vi "Results.vi"(0 "Code":dbl format="%#_12g", 5 "Voltage":dbl format="%#_12g", 11 "Error In":errorcluster, 12 "Slope":dbl format="%#_12g", 13 "Offset_Error":dbl format="%#_12g", 14 "Gain_error":dbl format="%#_12g") -> (15 "error out":errorcluster)   [LabVIEW 2019]
uses:
  common/Comman_nilesh/File_Write/Data_Logging.lvclass
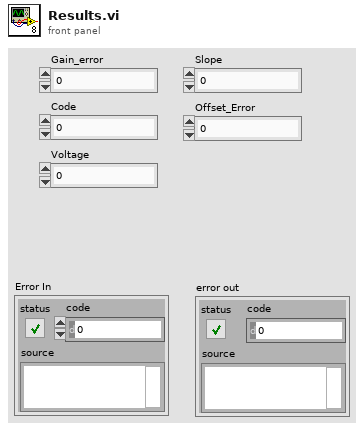
[diagram p1: front panel]
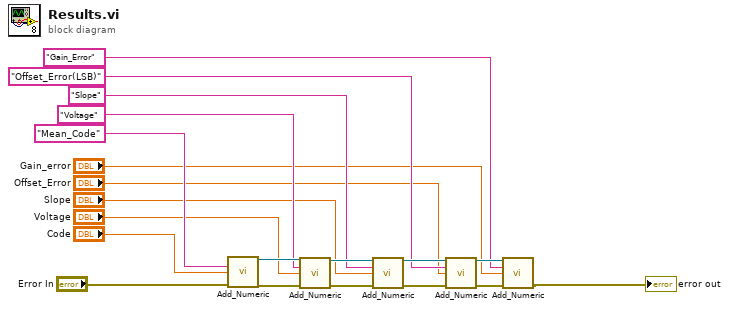
[diagram p0: block diagram]
diagram:
  n1 = call "Add_Numeric.vi"("Name"="Mean_Code", "Numeric_FC"="Code", "Error In"="Error In") -> ("Data_Logging.lvclass Out"=w14:refnum<class "Data_Logging.lvclass">, "error out"=w13:errorcluster)  [unwired: 11 in]
  n2 = call "Add_Numeric.vi"("Data_Logging.lvclass In"=w14, "Name"="Voltage", "Numeric_FC"="Voltage", "Error In"=w13) -> ("Data_Logging.lvclass Out"=w20:refnum<class "Data_Logging.lvclass">, "error out"=w19:errorcluster)  [unwired: 10 in]
  n3 = call "Add_Numeric.vi"("Data_Logging.lvclass In"=w20, "Name"="Slope", "Numeric_FC"="Slope", "Error In"=w19) -> ("Data_Logging.lvclass Out"=w18:refnum<class "Data_Logging.lvclass">, "error out"=w17:errorcluster)  [unwired: 10 in]
  n4 = call "Add_Numeric.vi"("Data_Logging.lvclass In"=w18, "Name"="Offset_Error(LSB)", "Numeric_FC"="Offset_Error", "Error In"=w17) -> ("Data_Logging.lvclass Out"=w16:refnum<class "Data_Logging.lvclass">, "error out"=w15:errorcluster)  [unwired: 10 in]
  n5 = call "Add_Numeric.vi"("Data_Logging.lvclass In"=w16, "Name"="Gain_Error", "Numeric_FC"="Gain_error", "Error In"=w15) -> ("error out"=→"error out":errorcluster)  [unwired: 10 in, 1 out]
